vi "Remove Above.vi"(7 "Y in":i32, 8 "Bottom in":i32[](array[numeric]), 9 "Top in":i32[](array[numeric]), 10 "Right in":i32[](array[numeric]), 11 "Left in":i32[](array[numeric])) -> (0 "Bottom out":i32[](array[numeric]), 1 "Top out":i32[](array[numeric]), 2 "Right out":i32[](array[numeric]), 3 "Left out":i32[](array[numeric]), 4 "empty?":bool)   [LabVIEW 2021, in "d14.lvlib"]
uses:
  d14.lvlib
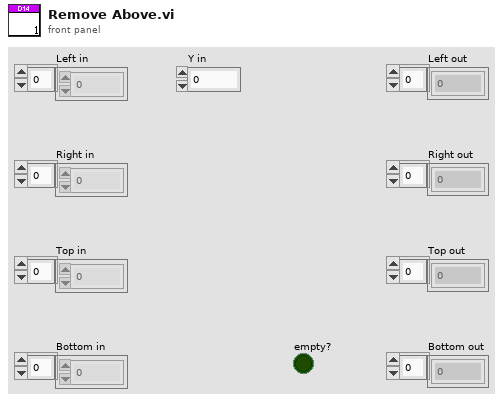
[diagram p1: front panel]
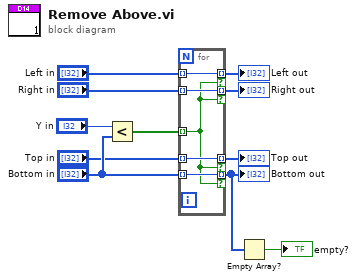
[diagram p0: block diagram]
diagram:
  n1 = Less?(x="Y in", y="Bottom in") -> (x < y?=w1:bool[])
  n2 = for {
    tunnel: w1 -> [w12] mode=indexing
    tunnel: "Top in" -> [w16] mode=indexing
    tunnel: "Bottom in" -> [w15] mode=indexing
    tunnel: [w15] -> w4 mode=indexing if=w12
    tunnel: [w16] -> w11 mode=indexing if=w12
    tunnel: "Left in" -> [w14] mode=indexing
    tunnel: [w14] -> w8 mode=indexing if=w12
    tunnel: [w13] -> w10 mode=indexing if=w12
    tunnel: "Right in" -> [w13] mode=indexing
  }
  "Bottom out" <- w4
  "Top out" <- w11
  "Right out" <- w10
  "Left out" <- w8
  n3 = Empty Array?(array=w4) -> (empty?=→"empty?":bool)
